vi "Main RLC.vi"() -> ()   [LabVIEW 2019]
uses:
  Types/Parameters Values Type.ctl
  Data Share Type.ctl
  <vilib>/picture/picture.llb/imagedata.ctl
  Types/Circuit Type Enum.ctl
panel:
  in  "Python file path":path=path "C:/Users/lukas/OneDrive/Desktop/LabView Projects/labview_methods.py"
  in  "Python Version":enum32{"2.7", "3.6"}(radio)
  in  "Select environment":enum32{"dev.", "demo.", ""}(radio)
  out "POST/PATCH Request error out":errorcluster
  out "Assigned attachments":string
  out "Updated formInput":string
  out "GET request error":errorcluster
  in  "Parameter Names":T1={"Vin"="Vin", "R"="R", "L"="L", "C"="C", "Series"="Series", "Parallel"="Parallel"}
  in  "Post Button":bool
  in  "Serial circuit fIlepath":path=path "C:/Users/lukas/OneDrive/Desktop/Refactored/series.png"
  in  "Parallel circuit fIlepath":path=path "C:/Users/lukas/OneDrive/Desktop/Refactored/parallel.png"
  in  "Save Button":bool
  out "Serial - Frequency Response Picture":picture
  out "Parallel - Frequency Response Picture":picture
  in  "Calculate Button":bool
  out "Parameters Values":T2
  in  "API Token":string="apitoken 3d0f3d54-6d52-4556-b227-557e3cfc9149:4f4ae2da-54ff-4843-ba38-552ad6772c0e"
  in  "DocId":string="LUK00004"
  in  "Get Button":bool
  in  "Close Button":bool
  # "1. GET request to receive filter parameters"
  # "2. Calculate Parallel/Serial circuits frequency responce"
  # "3. Save to file"
  # "4. POST/PUT requests to send images and update formInput"
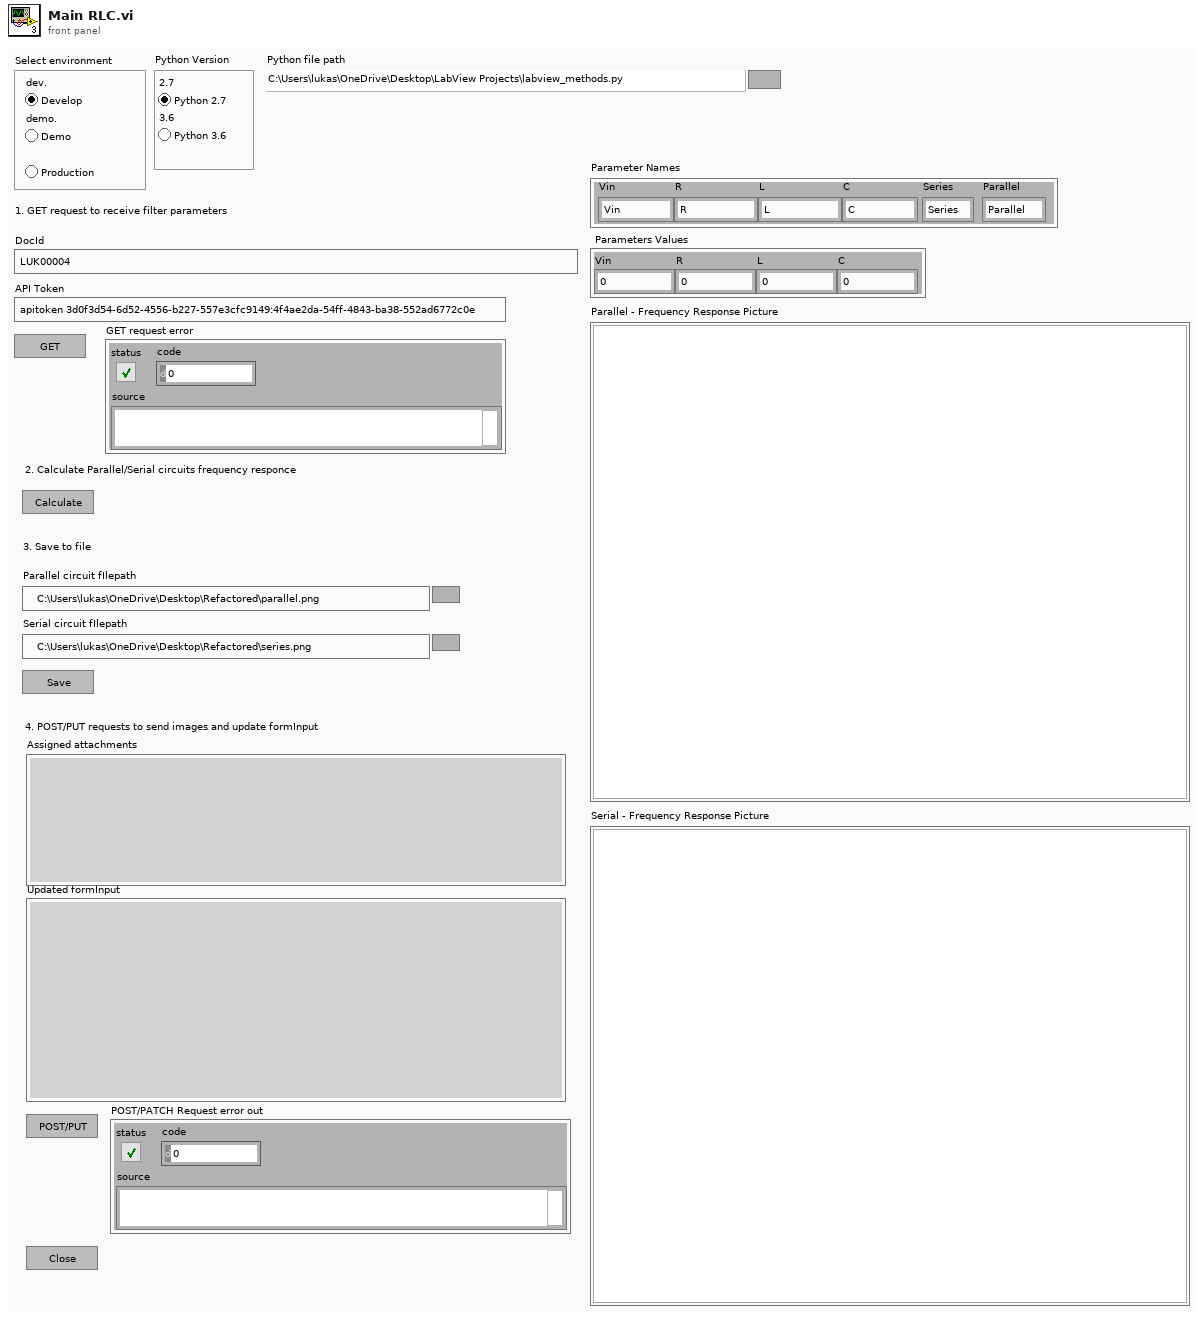
[diagram p1: front panel]
types:
  T1 = cluster{"Vin":string, "R":string, "L":string, "C":string, "Series":string, "Parallel":string}
  T2 = typedef "Parameters Values Type.ctl" = cluster{"Vin":dbl, "R":dbl, "L":dbl, "C":dbl}
  T3 = typedef "Data Share Type.ctl" = cluster{"Parallel Image Data":T4, "Serial Image Data":T4, "Parameters Values":T2, "Parallel circuit fIlepath":path, "Serial circuit fIlepath":path, "Document Id":string, "Parallel File Id":string, "Serial File Id":string, "Api Token":string, "Output Series XY":string, "Output Parallel XY":string, "FormInput Names":string, "FormInput Values":string, "Select environment":enum32{"dev.", "demo.", ""}, "Python Version":enum32{"2.7", "3.6"}, "Python file path":path}
  T4 = typedef "imagedata.ctl" = cluster{"image type":i32, "image depth":i32, "image":u8[], "mask":u8[], "colors":u32[], "Rectangle":cluster{"left":i16, "top":i16, "right":i16, "bottom":i16}}
  T5 = typedef "Circuit Type Enum.ctl" = enum16{"Parallel", "Serial"}
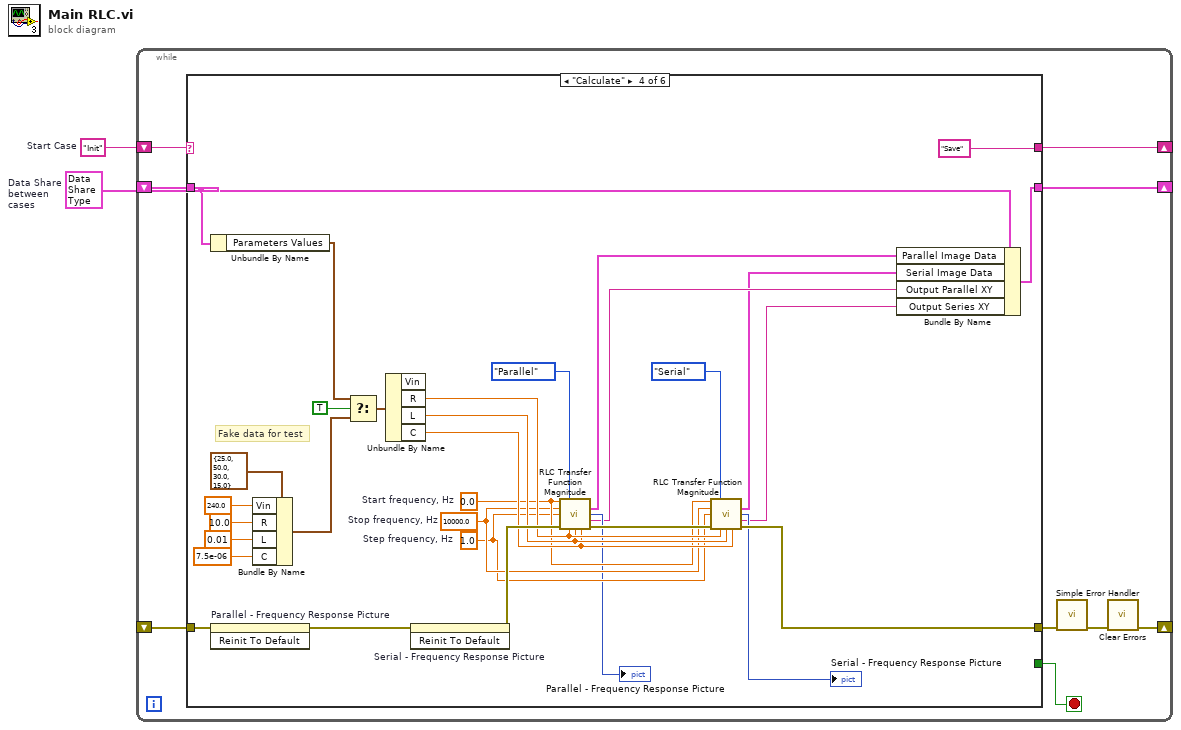
[diagram p0: block diagram]
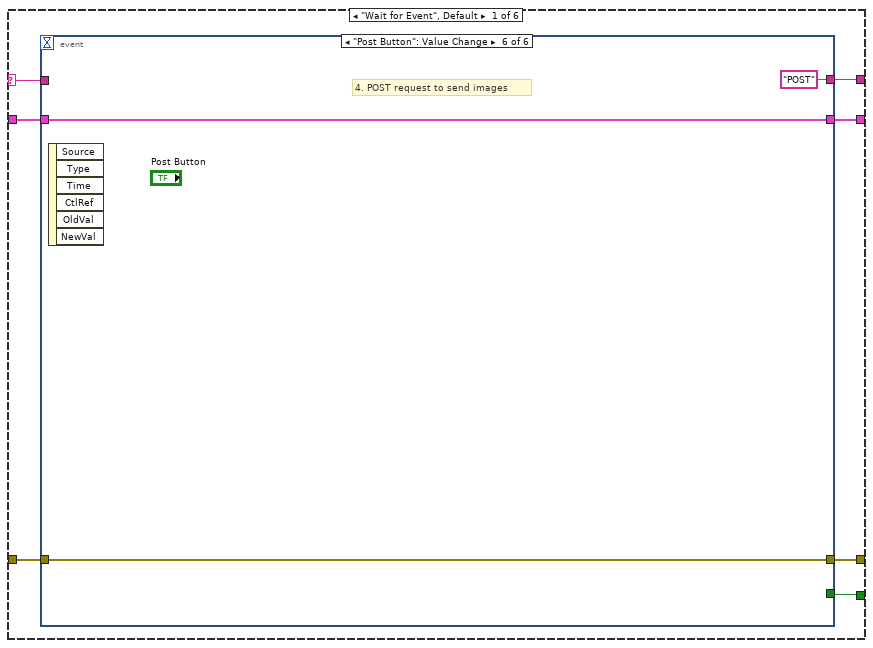
[diagram p2: hidden frame]
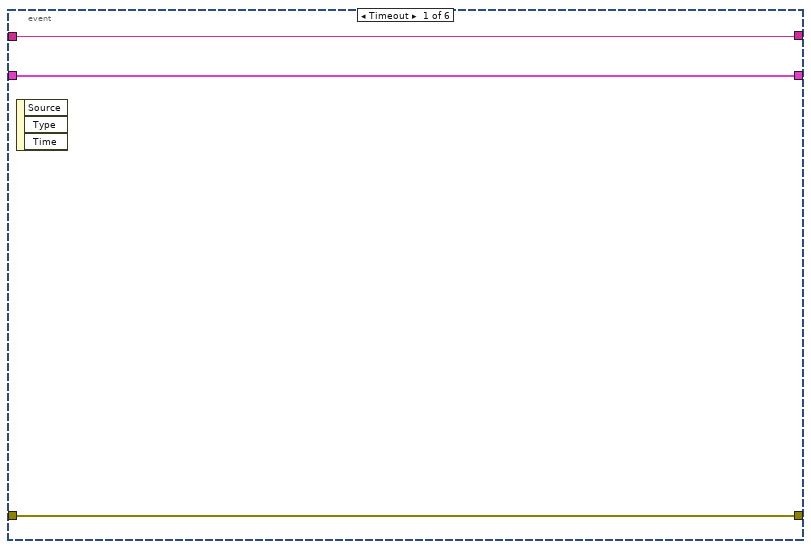
[diagram p3: hidden frame]
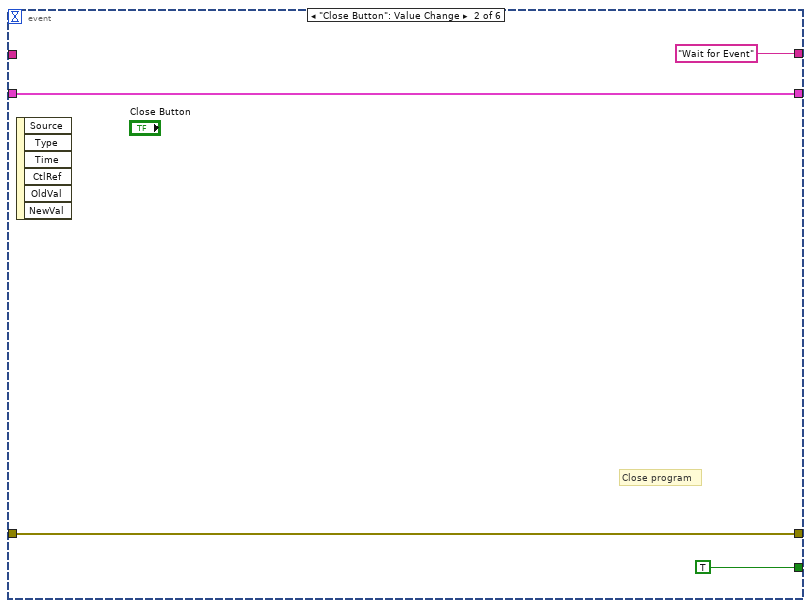
[diagram p4: hidden frame]
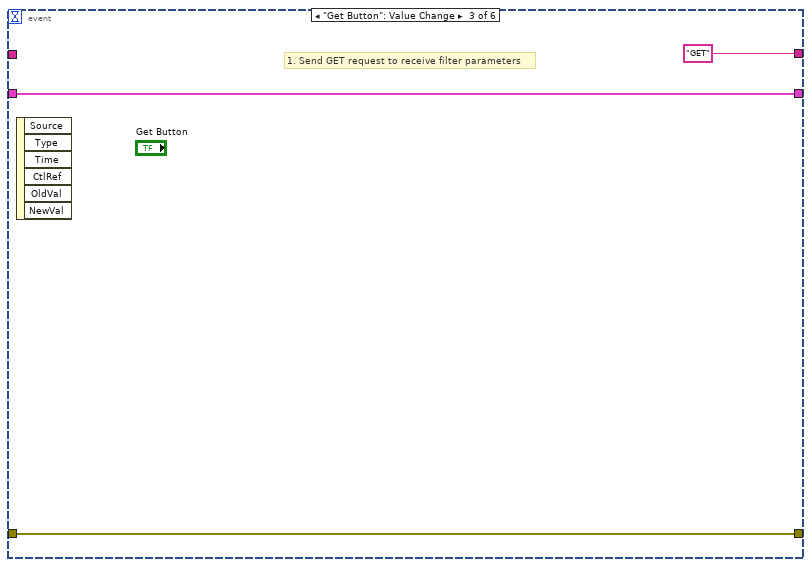
[diagram p5: hidden frame]
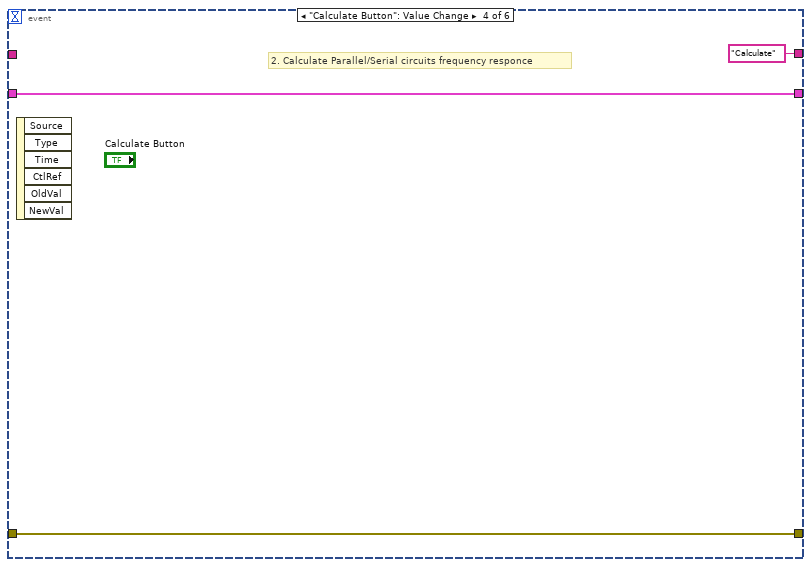
[diagram p6: hidden frame]
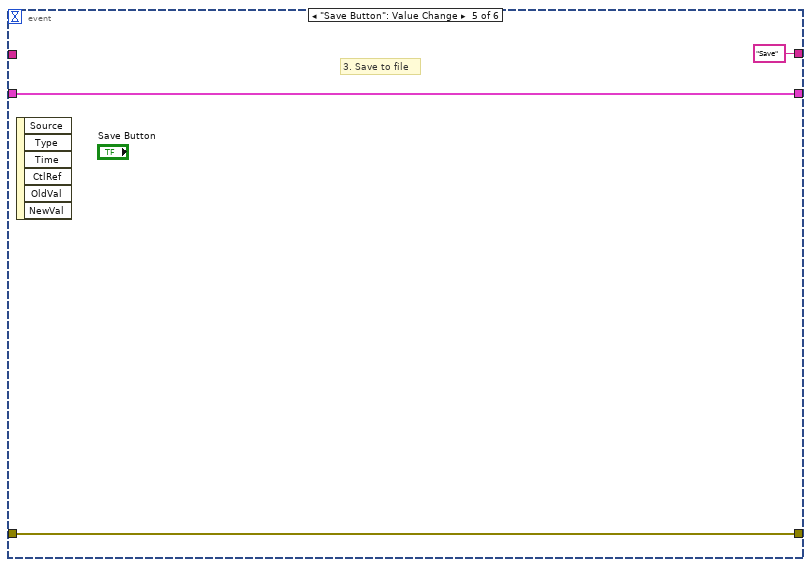
[diagram p7: hidden frame]
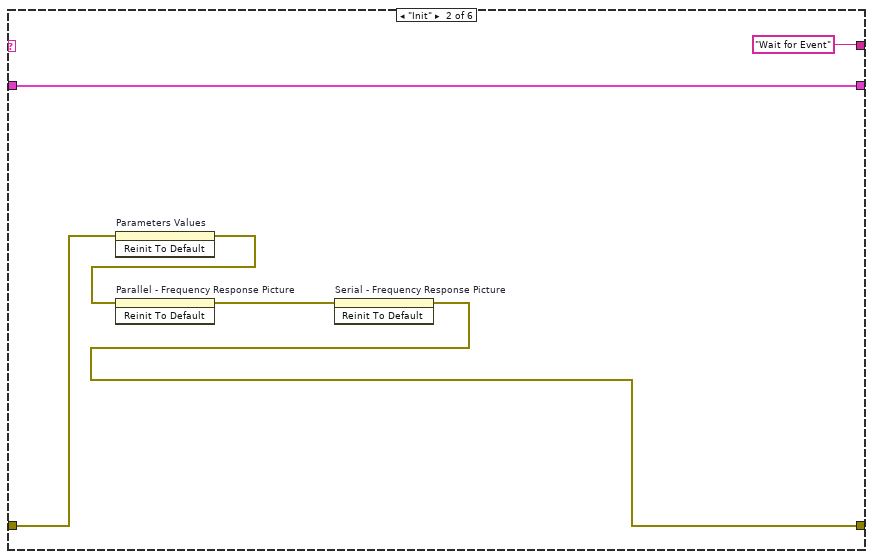
[diagram p8: hidden frame]
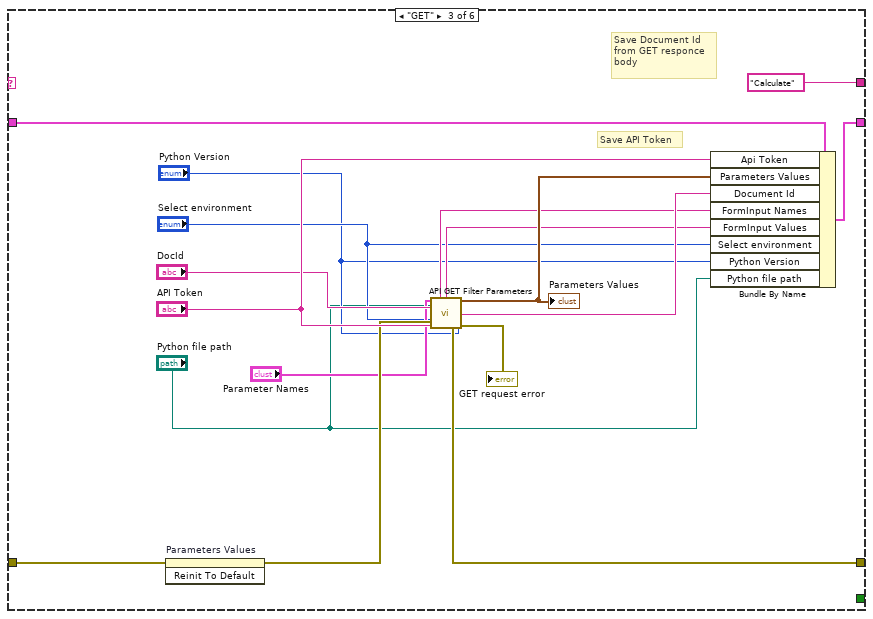
[diagram p9: hidden frame]
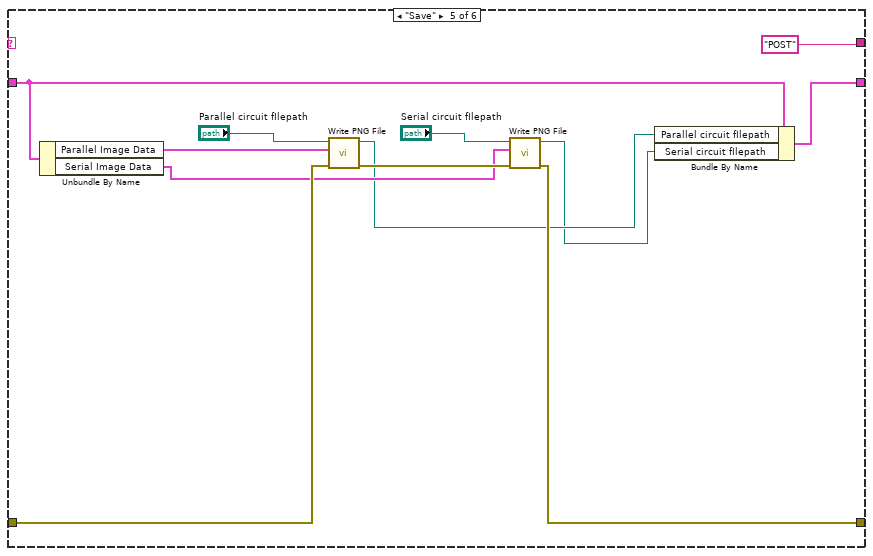
[diagram p10: hidden frame]
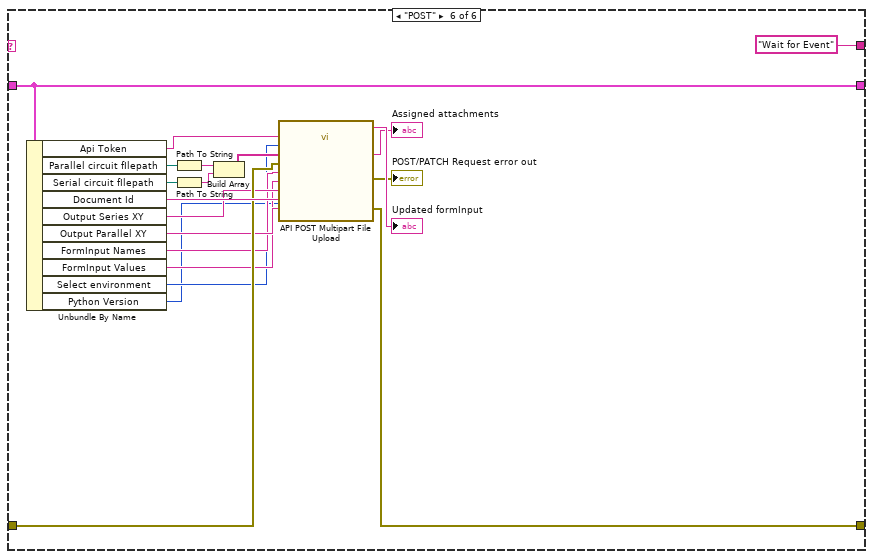
[diagram p11: hidden frame]
diagram:
  w1 = T3 {"Parallel Image Data"={"image type"=0, "image depth"=0, "image"=[], "mask"=[], "colors"=[], "Rectangle"={"left"=0, "top"=0, "right"=0, "bottom"=0}}, "Serial Image Data"={"image type"=0, "image depth"=0, "image"=[], "mask"=[], "colors"=[], "Rectangle"={"left"=0, "top"=0, "right"=0, "bottom"=0}}, "Parameters Values"={"Vin"=0.0, "R"=0.0, "L"=0.0, "C"=0.0}, "Parallel circuit fIlepath"=path "D:/upwork/Labview-REST-API/parallel.png", "Serial circuit fIlepath"=path "D:/upwork/Labview-REST-API/serial.png", "Document Id"="", "Parallel File Id"="", "Serial File Id"="", "Api Token"="", "Output Series XY"="", "Output Parallel XY"="", "FormInput Names"="", "FormInput Values"="", "Select environment"=enum."dev.", "Python Version"=enum."2.7", "Python file path"=path ""}  # Data Share between  cases
  w2 = "Init"  # Start Case
  n1 = while {
    shift-right: [w9] -> _
    shift-left: w2 -> [w11]
    shift-right: [w5] -> _
    shift-left: _ -> [w8]
    shift-right: [w3] -> _
    shift-left: w1 -> [w4]
    stop <- w10 stop-if-true
    n2 = case shown="\"Calculate\"" w11 {
      selector: w11 -> [w17 _ _ _ _ _]
      tunnel: [w18 _ _ _ _ _] -> w10
      tunnel: [w16 "Wait for Event" "Calculate" "Save" "POST" "Wait for Event"] -> w9
      tunnel: [w14 w38 w52 w75 w96 w121] -> w7
      tunnel: w8 -> [w15 w42 w59 w91 w100 w119]
      tunnel: w4 -> [w13 w40 w46 w80 w94 w113]
      tunnel: [w12 w40 w58 w79 w95 w113] -> w3
      frame "Wait for Event", Default {
        n3 = event shown="[5] \"Post Button\": Value Change" {
          selector: _ -> [_ _ _ _ _ _]
          dyn-events: _ -> [_ _ _ _ _ _]
          timeout: _ -> [_ _ _ _ _ _]
          tunnel: [_ TRUE _ _ _ _] -> w18
          tunnel: w17 -> [w21 _ _ _ _ _]
          tunnel: [w21 "Wait for Event" "GET" "Calculate" "Save" "POST"] -> w16
          tunnel: w15 -> [w20 w23 w27 w30 w32 w35]
          tunnel: [w20 w23 w27 w30 w32 w35] -> w14
          tunnel: w13 -> [w19 w22 w26 w29 w33 w36]
          tunnel: [w19 w22 w26 w29 w33 w36] -> w12
          event Timeout {
            n4 = event-data() -> ()  [unwired: 1 in, 3 out]
          }
          event "Close Button": Value Change {
            # "Close program"
            n5 = event-data() -> ()  [unwired: 1 in, 6 out]
          }
          event "Get Button": Value Change {
            # "1. Send GET request to receive filter parameters"
            n6 = event-data() -> ()  [unwired: 1 in, 6 out]
          }
          event "Calculate Button": Value Change {
            # "2. Calculate Parallel/Serial circuits frequency responce"
            n7 = event-data() -> ()  [unwired: 1 in, 6 out]
          }
          event "Save Button": Value Change {
            # "3. Save to file"
            n8 = event-data() -> ()  [unwired: 1 in, 6 out]
          }
          event "Post Button": Value Change {
            # "4. POST request to send images"
            n9 = event-data() -> ()  [unwired: 1 in, 6 out]
          }
        }
      }
      frame "Init" {
        n10 = invoke on="Parameters Values" class="Clust (strict)" method="Reinit To Default"(error in=w42) -> (error out=w39:errorcluster)  [unwired: 2 in, 2 out]
        n11 = invoke on="Parallel - Frequency Response Picture" class="Pict" method="Reinit To Default"(error in=w39) -> (error out=w41:errorcluster)  [unwired: 2 in, 2 out]
        n12 = invoke on="Serial - Frequency Response Picture" class="Pict" method="Reinit To Default"(error in=w41) -> (error out=w38:errorcluster)  [unwired: 2 in, 2 out]
      }
      frame "GET" {
        # "Save Document Id\nfrom GET responce\nbody"
        # "Save API Token"
        n13 = invoke on="Parameters Values" class="Clust (strict)" method="Reinit To Default"(error in=w59) -> (error out=w53:errorcluster)  [unwired: 2 in, 2 out]
        n14 = call "API GET Filter Parameters.vi"("Cluster"="Parameter Names", "Python file path"="Python file path", "docId"="DocId", "Select environment"="Select environment", "Python Version"="Python Version", "ApiToken"="API Token", "error in GET"=w53) -> ("GET RESPONSE (FromInput Names)"=w50:string, "GET RESPONSE (FormInput Values)"=w49:string, "Parameters Values"=w57:T2, "Document Revision Id"=w54:string, "GET error out"=w52:errorcluster, "GET request error"=→"GET request error":errorcluster)  [unwired: 3 in]
        "Parameters Values" <- w57
        n15 = Bundle By Name(cluster=w46, "Api Token"="API Token", "Parameters Values"=w57, "Document Id"=w54, "FormInput Names"=w50, "FormInput Values"=w49, "Select environment"="Select environment", "Python Version"="Python Version", "Python file path"="Python file path") -> (w58:T3)
      }
      frame "Calculate" {
        w69 = 1.0  # Step frequency, Hz
        w70 = 10000.0  # Stop frequency, Hz
        w71 = 0.0  # Start frequency, Hz
        # "Fake data for test"
        n16 = Unbundle By Name(w80) -> ("Parameters Values"=w81:T2)
        n17 = invoke on="Parallel - Frequency Response Picture" class="Pict" method="Reinit To Default"(error in=w91) -> (error out=w90:errorcluster)  [unwired: 2 in, 2 out]
        n18 = Bundle By Name(cluster=T2 {"Vin"=25.0, "R"=50.0, "L"=30.0, "C"=15.0} ("Parameters Values"), "Vin"=240.0, "R"=10.0, "L"=0.01, "C"=7.5e-06) -> (w84:T2)
        n19 = Select(t=w81, s=TRUE, f=w84) -> (s? t:f=w83:T2)
        n20 = Unbundle By Name(w83) -> ("R"=w74:dbl, "L"=w73:dbl, "C"=w72:dbl)  [unwired: 1 out]
        n21 = invoke on="Serial - Frequency Response Picture" class="Pict" method="Reinit To Default"(error in=w90) -> (error out=w77:errorcluster)  [unwired: 2 in, 2 out]
        n22 = call "RLC Transfer Function Magnitude.vi"("Start frequency, Hz"=w71, "Circuit Type"=Circuit_Type_Enum."Parallel" ("Circuit Type Enum"), "Stop frequency, Hz"=w70, "Step frequency, Hz"=w69, "error in (no error)"=w77, "R, Ohm"=w74, "L, H"=w73, "C, F"=w72) -> ("RLC Circuit Transfer function\n (magnitude) Image Data"=w62:T4, "RLC Circuit Transfer function (magnitude) Picture"=→"Parallel - Frequency Response Picture":picture, "JSON string"=w65:string, "error out"=w76:errorcluster)  [unwired: 3 in, 1 out]
        n23 = call "RLC Transfer Function Magnitude.vi"("Start frequency, Hz"=w71, "Circuit Type"=Circuit_Type_Enum."Serial" ("Circuit Type Enum"), "Stop frequency, Hz"=w70, "Step frequency, Hz"=w69, "error in (no error)"=w76, "R, Ohm"=w74, "L, H"=w73, "C, F"=w72) -> ("RLC Circuit Transfer function\n (magnitude) Image Data"=w63:T4, "RLC Circuit Transfer function (magnitude) Picture"=→"Serial - Frequency Response Picture":picture, "JSON string"=w64:string, "error out"=w75:errorcluster)  [unwired: 3 in, 1 out]
        n24 = Bundle By Name(cluster=w80, "Parallel Image Data"=w62, "Serial Image Data"=w63, "Output Parallel XY"=w65, "Output Series XY"=w64) -> (w79:T3)
      }
      frame "Save" {
        n25 = Unbundle By Name(w94) -> ("Parallel Image Data"=w101:T4, "Serial Image Data"=w97:T4)
        n26 = call <vilib>:"Write PNG File.vi"("error in (no error)"=w100, "image data"=w101, "path to PNG file"="Parallel circuit fIlepath") -> ("error out"=w99:errorcluster, "path"=w93:path)  [unwired: 7 in]
        n27 = call <vilib>:"Write PNG File.vi"("error in (no error)"=w99, "image data"=w97, "path to PNG file"="Serial circuit fIlepath") -> ("error out"=w96:errorcluster, "path"=w92:path)  [unwired: 7 in]
        n28 = Bundle By Name(cluster=w94, "Parallel circuit fIlepath"=w93, "Serial circuit fIlepath"=w92) -> (w95:T3)
      }
      frame "POST" {
        n29 = Unbundle By Name(w113) -> ("Api Token"=w122:string, "Parallel circuit fIlepath"=w117:path, "Serial circuit fIlepath"=w115:path, "Document Id"=w120:string, "Output Series XY"=w112:string, "Output Parallel XY"=w111:string, "FormInput Names"=w110:string, "FormInput Values"=w109:string, "Select environment"=w105:enum32{"dev.", "demo.", ""}, "Python Version"=w104:enum32{"2.7", "3.6"})
        n30 = Path To String(path=w117) -> (string=w116:string)
        n31 = Path To String(path=w115) -> (string=w114:string)
        n32 = Build Array(w116, w114) -> (w118:string[])
        n33 = call "API POST Multipart File Upload.vi"("DocumentRevisionId"=w120, "XY Parallel"=w111, "Python Version"=w104, "XY Series"=w112, "API Token"=w122, "Select environment"=w105, "Paths"=w118, "POST/PATCH error in (no error)"=w119, "FormInput Names"=w110, "FormInput Values"=w109) -> ("Updated formInput"=→"Updated formInput":string, "Assigned attachments"=→"Assigned attachments":string, "POST/PATCH Request error out"=→"POST/PATCH Request error out":errorcluster, "POST/PATCH error out"=w121:errorcluster)  [unwired: 2 in]
      }
    }
    n34 = call <vilib>:"Simple Error Handler.vi"("error in (no error)"=w7) -> ("error out"=w6:errorcluster)  [unwired: 4 in, 4 out]
    n35 = call <vilib>:"Clear Errors.vi"("error in (no error)"=w6) -> ("error out"=w5:errorcluster)  [unwired: 5 in, 1 out]
  }
